vi "Read File.vi"(8 "error in (no error)":errorcluster, 11 "Data.HDF5 Save in":refnum<class "Data.HDF5.lvclass">) -> (0 "error out":errorcluster, 3 "Data.HDF5 Save out":refnum<class "Data.HDF5.lvclass">)   [LabVIEW 2016, in "Data.HDF5.lvclass"]
uses:
  Data.HDF5.lvclass
  C:/user/patrick/git/LV-to-ITX/src/Data/Data.lvclass
  Data/Data.lvclass/Data.ctl
  Data/Data.lvclass
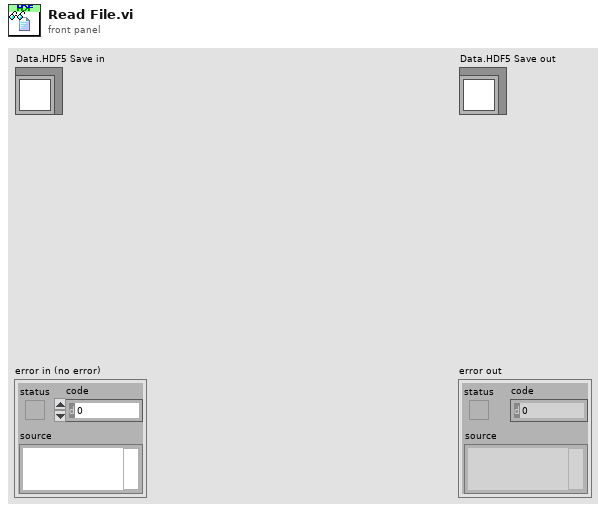
[diagram p1: front panel]
types:
  T1 = typedef "Data.lvclass/Dictionary--cluster.ctl" = cluster{"key":string, "value":variant}
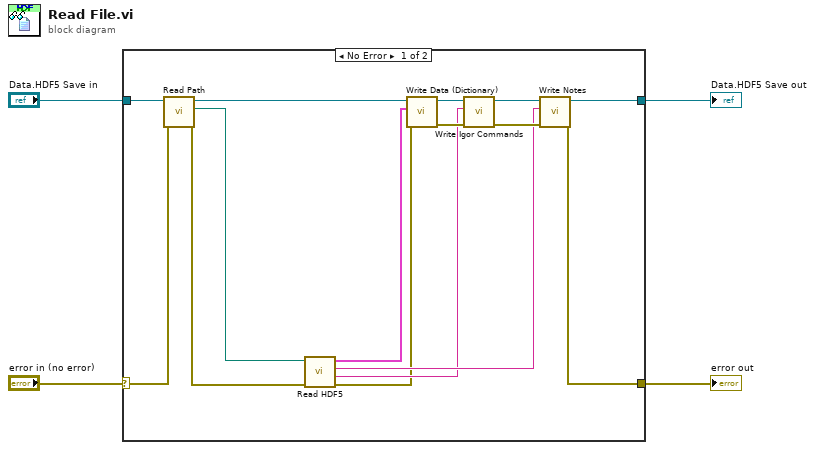
[diagram p0: block diagram]
diagram:
  n1 = case shown="No Error" "error in (no error)" {
    selector: "error in (no error)" -> [w11 w21]
    tunnel: "Data.HDF5 Save in" -> [w19 w20]
    tunnel: [w18 w20] -> w1
    tunnel: [w12 w21] -> w2
    frame No Error {
      n2 = call "Read Path.vi"("error in (no error)"=w11, "Data Save"=w19) -> ("error out"=w9:errorcluster, "Path"=w10:path, "Data Save out"=w15:refnum<class "Data.HDF5.lvclass">)  [unwired: 7 in]
      n3 = call "Read HDF5.vi"("error in (no error)"=w9, "path"=w10) -> ("error out"=w5:errorcluster, "Igor Commands"=w6:string, "Notes"=w7:string, "Data (Dictionary)"=w8:T1[])  [unwired: 6 in]
      n4 = call "Write Data (Dictionary).vi"("error in (no error)"=w5, "Data (Dictionary)"=w8, "Data Save"=w15) -> ("error out"=w14:errorcluster, "Data Save out"=w16:refnum<class "Data.HDF5.lvclass">)  [unwired: 7 in]
      n5 = call "Write Igor Commands.vi"("error in (no error)"=w14, "Igor Commands"=w6, "Data Save"=w16) -> ("error out"=w13:errorcluster, "Data Save out"=w17:refnum<class "Data.HDF5.lvclass">)  [unwired: 7 in]
      n6 = call "Write Notes.vi"("error in (no error)"=w13, "Notes"=w7, "Data Save"=w17) -> ("error out"=w12:errorcluster, "Data Save out"=w18:refnum<class "Data.HDF5.lvclass">)  [unwired: 7 in]
    }
    frame Error {
    }
  }
  "error out" <- w2
  "Data.HDF5 Save out" <- w1
